vi "ModeSelect.vi"(11 "Mode in":u16) -> (2 "Strings And Values []":T1, 3 "Mode out":u16)   [LabVIEW 2020]
uses:
  <vilib>/Utility/miscctls.llb/LVStringsAndValuesArrayTypeDef_U16.ctl
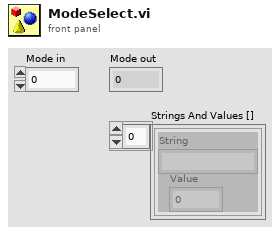
[diagram p1: front panel]
types:
  T1 = typedef "LVStringsAndValuesArrayTypeDef_U16.ctl" = cluster{"String":string, "Value":u16}[]
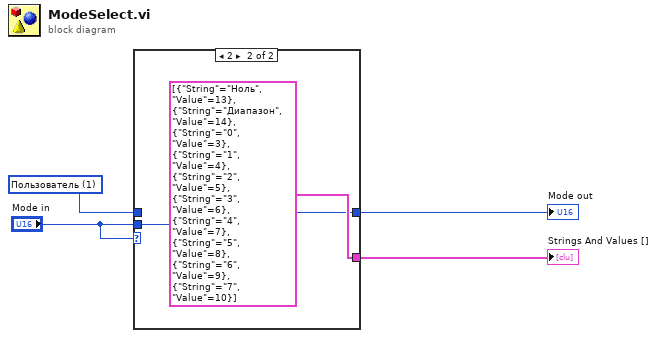
[diagram p0: block diagram]
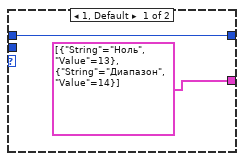
[diagram p2: hidden frame]
diagram:
  w4 = u16 1 items=["Пользователь"=1, "Инженер"=2, ""=0] ("Режим работы")
  n1 = case shown="2" "Mode in" {
    tunnel: [T1 [{"String"="Ноль", "Value"=13}, {"String"="Диапазон", "Value"=14}] ("Strings And Values []") T1 [{"String"="Ноль", "Value"=13}, {"String"="Диапазон", "Value"=14}, {"String"="0", "Value"=3}, {"String"="1", "Value"=4}, {"String"="2", "Value"=5}, {"String"="3", "Value"=6}, {"String"="4", "Value"=7}, {"String"="5", "Value"=8}, {"String"="6", "Value"=9}, {"String"="7", "Value"=10}] ("Strings And Values []")] -> w3
    tunnel: [w6 w7] -> w2
    tunnel: w4 -> [w6 _]
    tunnel: "Mode in" -> [_ w7]
    frame 1, Default {
    }
    frame 2 {
    }
  }
  "Strings And Values []" <- w3
  "Mode out" <- w2
